vi "AxisInit.vi"(1 "axis":i32) -> (0 "初始化成功成功？":bool)   [LabVIEW 2018]
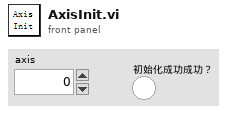
[diagram p1: front panel]
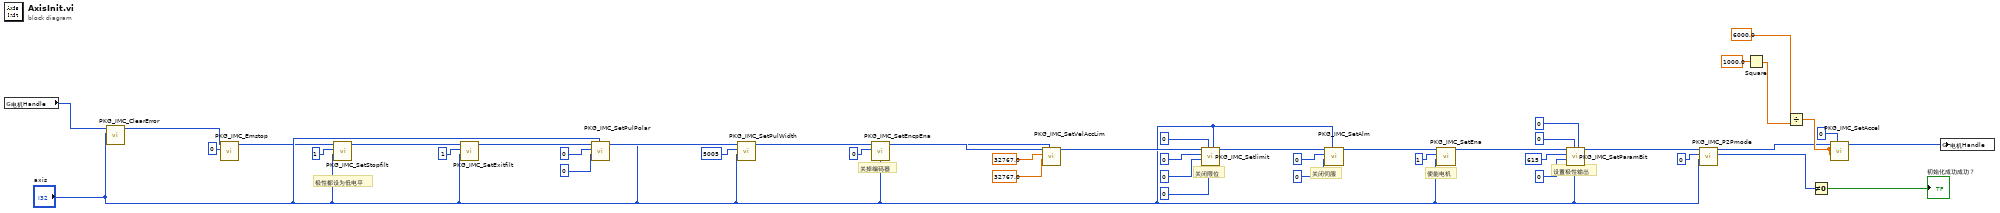
[diagram p0: block diagram]
diagram:
  # "设置极性输出"
  # "使能电机"
  # "关闭限位"
  # "关闭伺服"
  # "极性都设为低电平"
  # "关掉编码器"
  n1 = global read "参数.vi" "电机Handle"() -> (w34:u32)
  n2 = call "PKG_IMC_ClearError.vi"("axis"="axis", "Handle"=w34) -> ("Handle out"=w3:u32)  [unwired: 8 in, 1 out]
  n3 = call "PKG_IMC_Emstop.vi"("isStop"=0, "Handle"=w3) -> ("Handle out"=w2:u32)  [unwired: 8 in, 1 out]
  n4 = call "PKG_IMC_SetStopfilt.vi"("axis"="axis", "stop"=1, "handle"=w2) -> ("handle out"=w37:u32)  [unwired: 7 in, 1 out]
  n5 = call "PKG_IMC_SetExitfilt.vi"("axis"="axis", "exit"=1, "handle"=w37) -> ("handle out"=w35:u32)  [unwired: 7 in, 1 out]
  n6 = call "PKG_IMC_SetPulPolar.vi"("axis"="axis", "dir"=0, "pul"=0, "handle"=w35) -> ("handle out"=w41:u32)  [unwired: 6 in, 1 out]
  n7 = call "PKG_IMC_SetPulWidth.vi"("axis"="axis", "ns"=u32 5005, "handle"=w41) -> ("handle out"=w40:u32)  [unwired: 7 in, 1 out]
  n8 = call "PKG_IMC_SetEncpEna.vi"("axis"="axis", "ena"=0, "handle"=w40) -> ("handle out"=w16:u32)  [unwired: 7 in, 1 out]
  n9 = call "PKG_IMC_SetVelAccLim.vi"("axis"="axis", "acclim"=32767.0, "vellim"=32767.0, "handle"=w16) -> ("handle out"=w28:u32)  [unwired: 6 in, 1 out]
  n10 = call "PKG_IMC_Setlimit.vi"("axis"="axis", "nlimPolar"=0, "nlimEna"=0, "plimPolar"=0, "plimEna"=0, "handle"=w28) -> ("handle out"=w27:u32)  [unwired: 4 in, 1 out]
  n11 = call "PKG_IMC_SetAlm.vi"("axis"="axis", "polar"=0, "ena"=0, "handle"=w27) -> ("handle out"=w22:u32)  [unwired: 6 in, 1 out]
  n12 = call "PKG_IMC_SetEna.vi"("axis"="axis", "ena"=1, "handle"=w22) -> ("handle out"=w21:u32)  [unwired: 7 in, 1 out]
  n13 = call "PKG_IMC_SetParamBit.vi"("fifo"=0, "axis"="axis", "val"=i16 0, "bit"=i16 0, "paramloc"=i16 615, "Handle"=w21) -> ("Handle out"=w14:u32)  [unwired: 4 in, 1 out]
  n14 = call "PKG_IMC_P2Pmode.vi"("axis"="axis", "mode"=0, "handle"=w14) -> ("function return"=w12:i32, "handle out"=w5:u32)  [unwired: 7 in]
  n15 = Square(x=1000.0) -> (x^2=w8:dbl)
  n16 = Divide(x=6000.0 ("accel"), y=w8) -> (x/y=w7:dbl)
  n17 = Not Equal To 0?(x=w12) -> (x != 0?=→"初始化成功成功？":bool)
  n18 = call "PKG_IMC_SetAccel.vi"("axis"=0, "decel"=w7, "accel"=w7, "handle"=w5) -> ("handle out"=w4:u32)  [unwired: 6 in, 1 out]
  n19 = global write "参数.vi" "电机Handle"(w4) -> ()
